vi "TCP handler.vi"(9 "remote port":u16, 10 "remote address":string, 11 "connection ID":refnum<k5>) -> ()   [LabVIEW 2014, in "AMC.lvlib"]
uses:
  AMC.lvlib
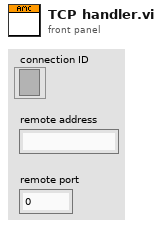
[diagram p1: front panel]
types:
  T1 = typedef "AMC.lvlib/Message.ctl" = cluster{"name":string, "value":string, "attributes":T2, "receiver host":string, "receiver process":string, "source host":string, "source process":string, "priority message":bool, "acknowledge message":bool}
  T2 = typedef "Tools_KeyedArray.lvlib/KeyedArray.ctl" = cluster{"keys":string[], "values":string[]}
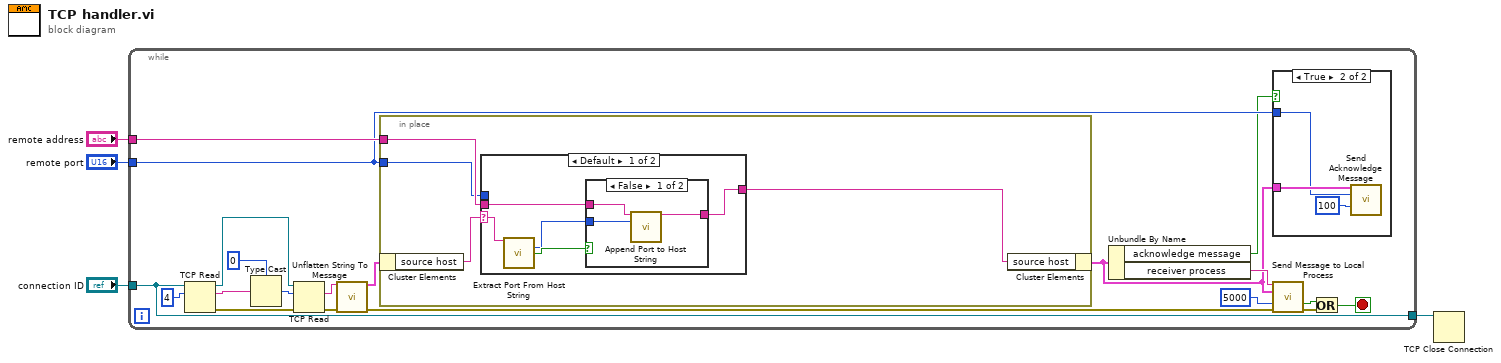
[diagram p0: block diagram]
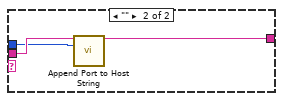
[diagram p4: hidden frame]
diagram:
  n1 = while {
    tunnel: "connection ID" -> [w8]
    tunnel: "remote port" -> [w7]
    tunnel: "remote address" -> [w15]
    tunnel: [w8] -> w1
    stop <- w9 stop-if-true
    n2 = TCP Read(connection ID=w8, bytes to read=4) -> (connection ID out=w21:refnum<k5>, data out=w23:string, error out=w19:errorcluster)  [unwired: 3 in]
    n3 = Type Cast(type=0 ("bytes to read"), x=w23) -> (*(type *) &x=w20:i32)
    n4 = TCP Read(connection ID=w21, bytes to read=w20, error in (no error)=w19) -> (data out=w18:string, error out=w17:errorcluster)  [unwired: 2 in, 1 out]
    n5 = call "Unflatten String To Message.vi"("message string"=w18, "error in"=w17) -> ("message"=w16:T1, "error out"=w12:errorcluster)  [unwired: 12 in]
    n6 = in-place {
      in-place-border: w7 -> [w29]
      in-place-border: w15 -> [w30]
      n7 = in-place-cluster #1(w16) -> ("source host"=w31:string)
      n8 = case shown="Default" w31 {
        selector: w31 -> [w36 _]
        tunnel: w30 -> [w34 w43]
        tunnel: w29 -> [_ w42]
        tunnel: [w33 w41] -> w28
        frame Default {
          n9 = call "Extract Port From Host String.vi"("host in"=w36) -> ("port"=w32:u16, "found?"=w35:bool)  [unwired: 12 in, 1 out]
          n10 = case shown="False" w35 {
            tunnel: w34 -> [w39 w40]
            tunnel: [w38 w40] -> w33
            tunnel: w32 -> [w37 _]
            frame False {
              n11 = call "Append Port to Host String.vi"("host in"=w39, "port"=w37) -> ("host out"=w38:string)  [unwired: 13 in]
            }
            frame True {
            }
          }
        }
        frame "" {
          n12 = call "Append Port to Host String.vi"("host in"=w43, "port"=w42) -> ("host out"=w41:string)  [unwired: 13 in]
        }
      }
      n13 = in-place-cluster #1("source host"=w28) -> (w5:T1)
    }
    n14 = Unbundle By Name(w5) -> ("acknowledge message"=w6:bool, "receiver process"=w14:string)
    n15 = case shown="True" w6 {
      tunnel: w5 -> [_ w27]
      tunnel: w7 -> [_ w26]
      frame False {
      }
      frame True {
        n16 = call "Send Acknowledge Message.vi"("received message"=w27, "receiver port"=w26, "timeout"=100) -> ()  [unwired: 11 in, 2 out]
      }
    }
    n17 = call "Send Message to Local Process.vi"("process name"=w14, "message"=w5, "timeout (-1 ms)"=5000, "error in"=w12) -> ("timed out?"=w11:bool, "error out"=w10:errorcluster)  [unwired: 10 in]
    n18 = Or(x=w11, y=w10) -> (x .or. y?=w9:bool)
  }
  n19 = TCP Close Connection(connection ID=w1) -> ()  [unwired: 2 in, 2 out]
